vi "Fetch RJDJ Measurement.vi"(0 "VISA resource name":refnum<visa-resource-name>, 11 "error in (no error)":errorcluster) -> (1 "BUJ":T2, 2 "Misc":T1, 3 "TJ":T2, 4 "VISA resource name out":refnum<visa-resource-name>, 6 "RJ":T2, 8 "DJ":T2, 10 "PJ":T3, 12 "DDJ":T2, 13 "DCD":cluster{"Result":dbl, "State":i32}, 14 "ISI":T2, 15 "error out":errorcluster)   [LabVIEW 2013, in "Agilent 90000 Series.lvlib"]
doc: "Returns the results of the RJDJ Jitter measurement.\n\nNotes:\n\n(1) You must configure the appropriate reference levels before you call this VI to take measurement.\n\n(2) This VI does not check the instrument status. Typically, you call this VI only in a sequence of calls to other low-level driver VIs. The sequence performs one operation. You use the low-level VIs to optimize one or more aspects of interaction with the instrument. If you want to check the instrument status, call the Error-Query VI at the conclusion of the sequence."
uses:
  Agilent 90000 Series.lvlib
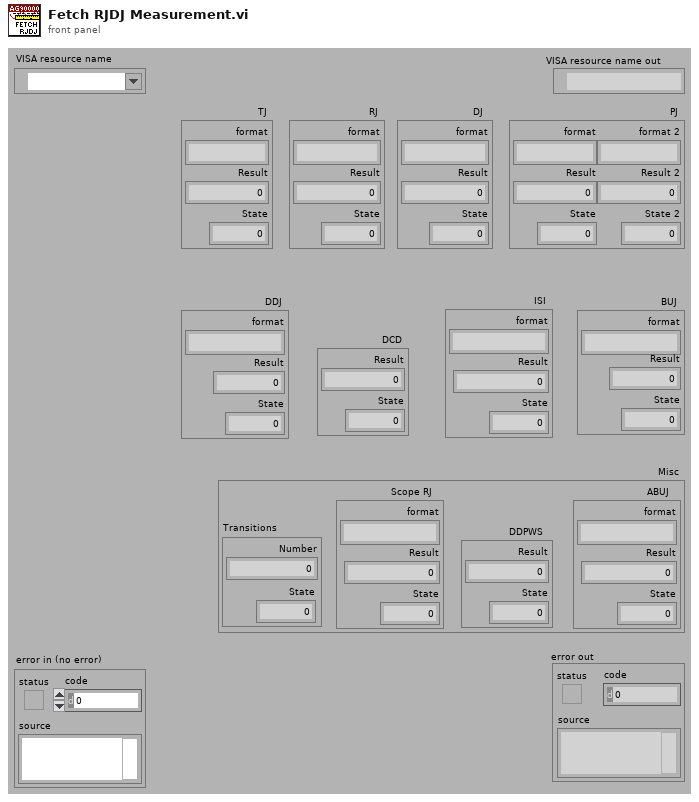
[diagram p1: front panel]
types:
  T1 = cluster{"Transitions":cluster{"Number":dbl, "State":i32}, "Scope RJ":cluster{"format":string, "Result":dbl, "State":i32}, "DDPWS":cluster{"Result":dbl, "State":i32}, "ABUJ":cluster{"format":string, "Result":dbl, "State":i32}}
  T2 = cluster{"format":string, "Result":dbl, "State":i32}
  T3 = cluster{"format":string, "Result":dbl, "State":i32, "format 2":string, "Result 2":dbl, "State 2":i32}
  T4 = cluster{cluster{dbl, i32}, cluster{string, dbl, i32}, cluster{dbl, i32}, cluster{string, dbl, i32}}
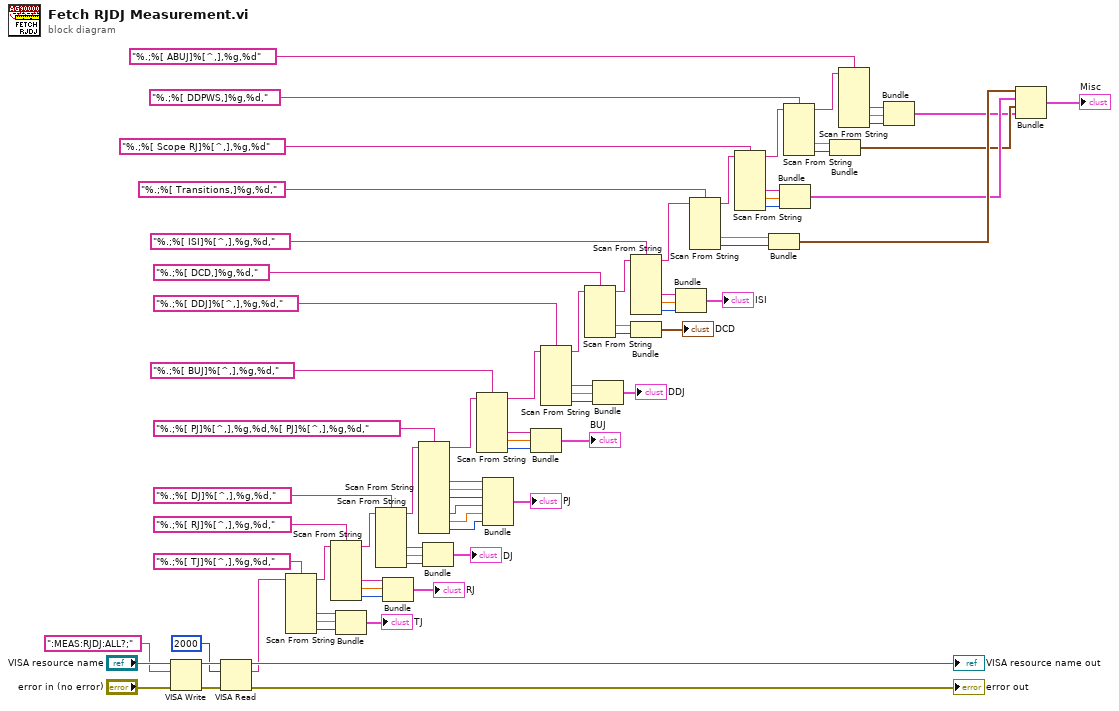
[diagram p0: block diagram]
diagram:
  n1 = VISA Write(VISA resource name="VISA resource name", write buffer=":MEAS:RJDJ:ALL?;", error in (no error)="error in (no error)") -> (VISA resource name out=w78:refnum<visa-resource-name>, error out=w77:errorcluster)  [unwired: 1 out]
  n2 = VISA Read(VISA resource name=w78, byte count=u32 2000, error in (no error)=w77) -> (VISA resource name out=→"VISA resource name out":refnum<visa-resource-name>, read buffer=w32:string, error out=→"error out":errorcluster)  [unwired: 1 out]
  n3 = Scan From String(format string="%.;%[ TJ]%[^,],%g,%d,", input string=w32) -> (remaining string=w70:string, output 2=w61:string, output 3=w60:dbl, output 4=w59:i32)  [unwired: 2 in, 7 out]
  n4 = Scan From String(format string="%.;%[ RJ]%[^,],%g,%d,", input string=w70) -> (remaining string=w73:string, output 2=w57:string, output 3=w56:dbl, output 4=w55:i32)  [unwired: 2 in, 7 out]
  n5 = Bundle(w61, w60, w59) -> (→"TJ":cluster{string, dbl, i32})  [unwired: 1 out]
  n6 = Scan From String(format string="%.;%[ DJ]%[^,],%g,%d,", input string=w73) -> (remaining string=w72:string, output 2=w54:string, output 3=w53:dbl, output 4=w52:i32)  [unwired: 2 in, 7 out]
  n7 = Bundle(w57, w56, w55) -> (→"RJ":cluster{string, dbl, i32})  [unwired: 1 out]
  n8 = Scan From String(format string="%.;%[ PJ]%[^,],%g,%d,%[ PJ]%[^,],%g,%d,", input string=w72) -> (remaining string=w30:string, output 2=w50:string, output 3=w49:dbl, output 4=w48:i32, output 6=w47:string, output 7=w46:dbl, output 8=w45:i32)  [unwired: 2 in, 12 out]
  n9 = Bundle(w54, w53, w52) -> (→"DJ":cluster{string, dbl, i32})  [unwired: 1 out]
  n10 = Scan From String(format string="%.;%[ BUJ]%[^,],%g,%d,", input string=w30) -> (remaining string=w24:string, output 2=w27:string, output 3=w26:dbl, output 4=w25:i32)  [unwired: 2 in, 7 out]
  n11 = Bundle(w50, w49, w48, w47, w46, w45) -> (→"PJ":cluster{string, dbl, i32, string, dbl, i32})  [unwired: 1 out]
  n12 = Bundle(w27, w26, w25) -> (→"BUJ":cluster{string, dbl, i32})  [unwired: 1 out]
  n13 = Scan From String(format string="%.;%[ DDJ]%[^,],%g,%d,", input string=w24) -> (remaining string=w71:string, output 2=w43:string, output 3=w42:dbl, output 4=w41:i32)  [unwired: 2 in, 7 out]
  n14 = Scan From String(format string="%.;%[ DCD,]%g,%d,", input string=w71) -> (remaining string=w69:string, output 2=w39:dbl, output 3=w38:i32)  [unwired: 2 in, 6 out]
  n15 = Bundle(w43, w42, w41) -> (→"DDJ":cluster{string, dbl, i32})  [unwired: 1 out]
  n16 = Scan From String(format string="%.;%[ ISI]%[^,],%g,%d,", input string=w69) -> (remaining string=w23:string, output 2=w36:string, output 3=w35:dbl, output 4=w34:i32)  [unwired: 2 in, 7 out]
  n17 = Bundle(w39, w38) -> (→"DCD":cluster{dbl, i32})  [unwired: 1 out]
  n18 = Bundle(w36, w35, w34) -> (→"ISI":cluster{string, dbl, i32})  [unwired: 1 out]
  n19 = Scan From String(format string="%.;%[ Transitions,]%g,%d,", input string=w23) -> (remaining string=w12:string, output 2=w19:dbl, output 3=w20:i32)  [unwired: 2 in, 6 out]
  n20 = Scan From String(format string="%.;%[ Scope RJ]%[^,],%g,%d", input string=w12) -> (remaining string=w11:string, output 2=w16:string, output 3=w15:dbl, output 4=w14:i32)  [unwired: 2 in, 7 out]
  n21 = Bundle(w19, w20) -> (w18:cluster{dbl, i32})  [unwired: 1 out]
  n22 = Bundle(w16, w15, w14) -> (w13:cluster{string, dbl, i32})  [unwired: 1 out]
  n23 = Scan From String(format string="%.;%[ DDPWS,]%g,%d,", input string=w11) -> (remaining string=w6:string, output 2=w9:dbl, output 3=w8:i32)  [unwired: 2 in, 6 out]
  n24 = Bundle(w9, w8) -> (w7:cluster{dbl, i32})  [unwired: 1 out]
  n25 = Scan From String(format string="%.;%[ ABUJ]%[^,],%g,%d", input string=w6) -> (output 2=w4:string, output 3=w3:dbl, output 4=w2:i32)  [unwired: 2 in, 8 out]
  n26 = Bundle(w4, w3, w2) -> (w1:cluster{string, dbl, i32})  [unwired: 1 out]
  n27 = Bundle(w18, w13, w7, w1) -> (→"Misc":T4)  [unwired: 1 out]
